vi "Close.vi"(7 "PTI":T1 {"Mono 2"."Flow Control" items=["1.0"=10, "1.5"=15, "2.0"=20]; "Mono 2"."Stop Bits" items=["None", "Odd", "Even", "Mark", "Space"]; "Mono 2"."Parity" items=["None", "Odd", "Even", "Mark", "Space"]; "Mono 1"."Flow Control" items=["1.0"=10, "1.5"=15, "2.0"=20]; "Mono 1"."Stop Bits" items=["None", "Odd", "Even", "Mark", "Space"]; "Mono 1"."Parity" items=["None", "Odd", "Even", "Mark", "Space"]}, 8 "error in (no error)":errorcluster) -> (0 "error out":errorcluster)   [LabVIEW 2017, in "Monochromator.lvlib" / "PTI.lvlib"]
uses:
  PTI.lvlib
  Controls/Params.ctl
  Controls/VISA parameters.ctl
  Serial comms/Serial comms.lvlib
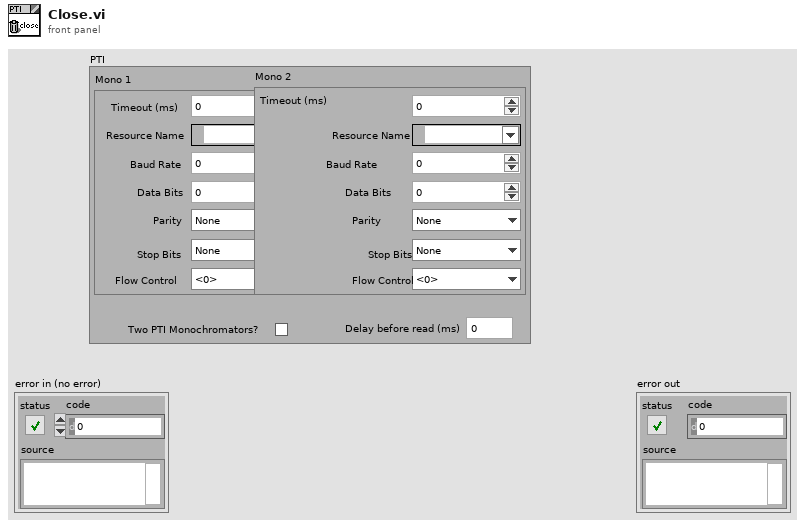
[diagram p1: front panel]
types:
  T1 = typedef "Monochromator.lvlib/PTI.lvlib/Params.ctl" = cluster{"Delay before read (ms)":u32, "Mono 1":T2, "Mono 2":T2, "Two PTI Monochromators?":bool}
  T2 = typedef "Serial comms.lvlib/VISA parameters.ctl" = cluster{"Timeout (ms)":u32, "Resource Name":refnum<visa-resource-name>, "Baud Rate":u32, "Data Bits":u16, "Parity":u16, "Stop Bits":u16, "Flow Control":u16}
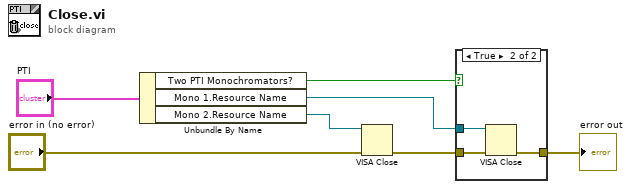
[diagram p0: block diagram]
diagram:
  n1 = Unbundle By Name("PTI") -> ("Two PTI Monochromators?"=w1:bool, "Mono 1.Resource Name"=w7:refnum<visa-resource-name>, "Mono 2.Resource Name"=w6:refnum<visa-resource-name>)
  n2 = VISA Close(VISA resource name=w6, error in (no error)="error in (no error)") -> (error out=w5:errorcluster)
  n3 = case shown="True" w1 {
    tunnel: w7 -> [_ w11]
    tunnel: w5 -> [w8 w10]
    tunnel: [w8 w9] -> w3
    frame False {
    }
    frame True {
      n4 = VISA Close(VISA resource name=w11, error in (no error)=w10) -> (error out=w9:errorcluster)
    }
  }
  "error out" <- w3
